vi "Image Processing.vi"(0 "File Path":path=path "C:/General AFM lithography program/Sample.ibw", 1 "Lithography Information":T2(array[cluster])=array7x3944[27608 elements], 2 "Crop?":bool, 3 "Crop Data":T3, 4 "Angle (degrees)":dbl, 5 "error in (no error)":errorcluster, 6 "Size":cluster{"Width":dbl, "Height":dbl}={"Width"=40.0, "Height"=40.0}, 7 "Page":i32=1, 11 "Resolution":i32=1024) -> (14 "Image Out":T4(plugin-control), 15 "Offset":T1={"X Offset (µm)"=-1.2812, "Y Offset (µm)"=5.2969}, 16 "Sample Size":cluster{"Width (µm)":dbl, "Height (µm)":dbl}={"Width (µm)"=40.0, "Height (µm)"=40.0}, 19 "error out":errorcluster)   [LabVIEW 2013]
uses:
  <vilib>/vision/NI_Vision_Development_Module.lvlib
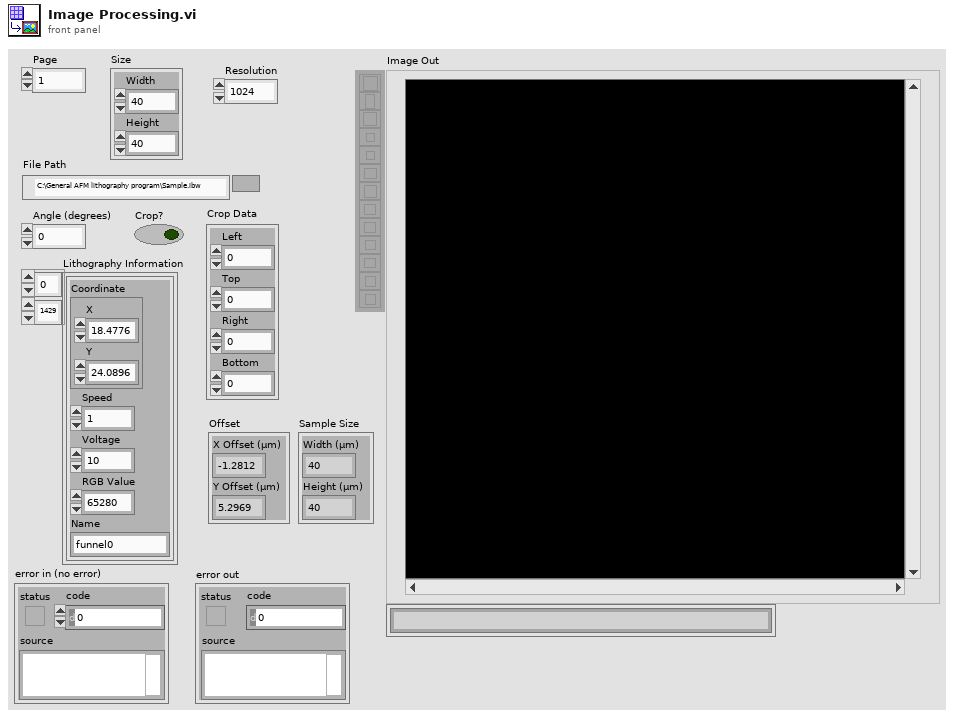
[diagram p1: front panel]
types:
  T1 = cluster{"X Offset (µm)":dbl, "Y Offset (µm)":dbl}
  T2 = cluster{"Coordinate":cluster{"X":dbl, "Y":dbl}, "Speed":dbl, "Voltage":dbl, "RGB Value":i32, "Name":string}[][]
  T3 = cluster{"Left":dbl, "Top":dbl, "Right":dbl, "Bottom":dbl}
  T4 = typedef "IMAQ Image.ctl" = refnum<image>
  T5 = typedef "Image Type" = u32
  T6 = cluster{"Coordinate":cluster{"X":dbl, "Y":dbl}, "Speed":dbl, "Voltage":dbl, "RGB Value":i32, "Name":string}
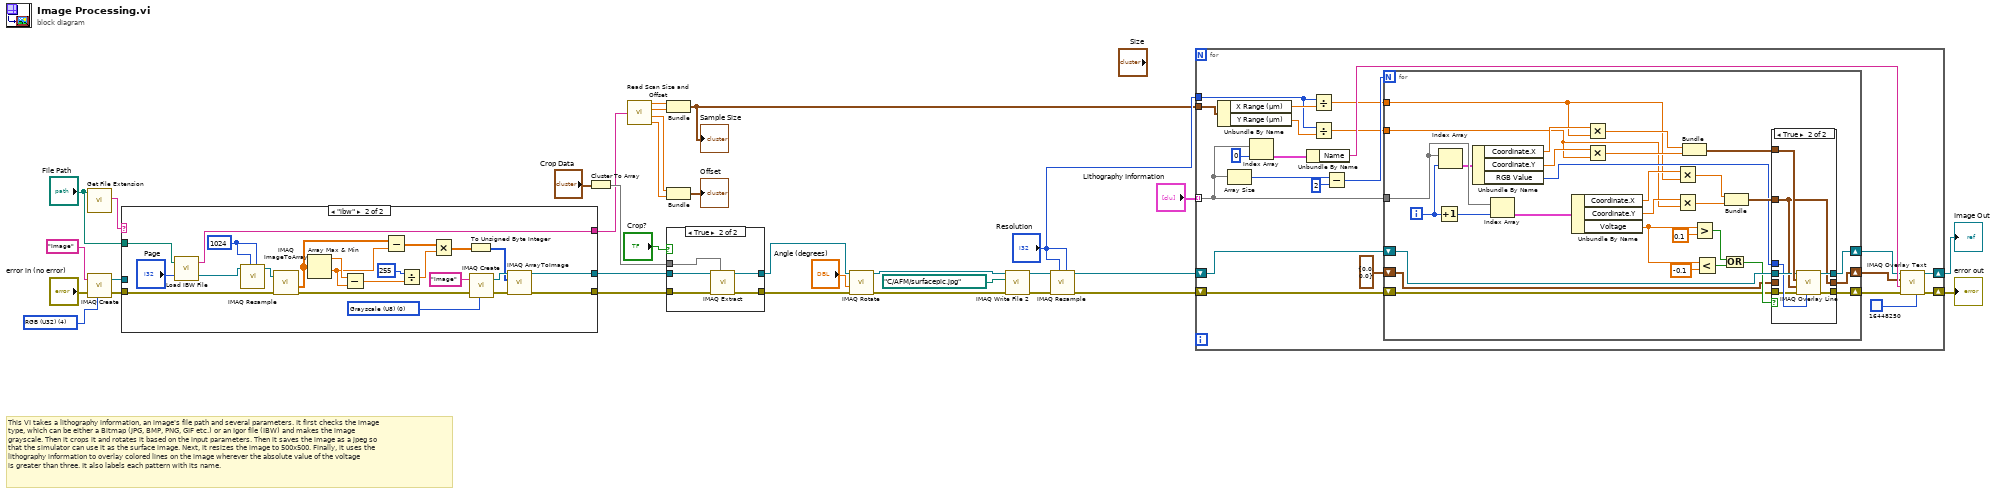
[diagram p0: block diagram]
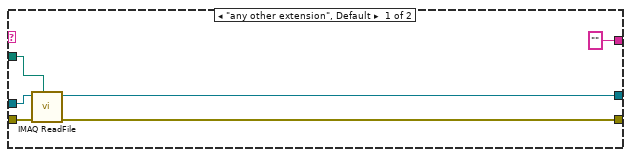
[diagram p2: hidden frame]
diagram:
  w32 = T5 4 items=["Grayscale (U8)", "Grayscale (I16)", "Grayscale (SGL)", "Complex (CSG)", "RGB (U32)", "HSL (U32)", "RGB (U64)", "Grayscale (U16)"] ("Image Type")
  # "This VI takes a lithography information, an image's file path and several parameters. It first checks the image \ntype, which can be either a Bitmap (JPG, BMP, PNG, GIF etc.) or an Igor file (IBW) and makes the image \ngrayscale. Then it crops it and rotates it based on the input parameters. Then it saves the image as a jpeg so \nthat the simulator can use it as the surface image. Next, it resizes the image to 500x500. Finally, it uses the \nlithography information to overlay colored lines on the image wherever the absolute value of the voltage \nis greater than three. It also labels each pattern with its name."
  n1 = call <vilib>:"Get File Extension.vi"("file"="File Path") -> ("lowercase file extension"=w19:string)  [unwired: 7 in, 3 out]
  n2 = call "IMAQ Create"("Image Name"="Image", "Image Type"=w32, "error in (no error)"="error in (no error)") -> ("New Image"=w31:T4, "error out"=w30:errorcluster)  [unwired: 2 in]
  n3 = case shown="\"ibw\"" w19 {
    tunnel: w31 -> [w39 _]
    tunnel: w30 -> [w38 w60]
    tunnel: [w37 w53] -> w29
    tunnel: [w36 w52] -> w28
    tunnel: "File Path" -> [w35 w62]
    tunnel: ["" ("Wave Note") w40] -> w8
    frame "any other extension", Default {
      n4 = call "IMAQ ReadFile"("File Path"=w35, "error in (no error)"=w38, "Image"=w39) -> ("error out"=w36:errorcluster, "Image Out"=w37:T4)  [unwired: 4 in, 3 out]
    }
    frame "ibw" {
      w50 = 1024 ("Y Resolution")
      w57 = T5 0 items=["Grayscale (U8)", "Grayscale (I16)", "Grayscale (SGL)", "Complex (CSG)", "RGB (U32)", "HSL (U32)", "RGB (U64)", "Grayscale (U16)"] ("Image Type")
      n5 = call "Load IBW File.vi"("Page"="Page", "file path (dialog if empty)"=w62) -> ("Image"=w49:T4, "Wave Note"=w40:string)
      n6 = call "IMAQ Resample"("X Resolution"=w50, "Y Resolution"=w50, "Image Src"=w49) -> ("Image Dst Out"=w48:T4)  [unwired: 7 in, 1 out]
      n7 = call "IMAQ ImageToArray"("error in (no error)"=w60, "Image"=w48) -> ("Image Pixels (Float)"=w59:sgl[][], "error out"=w54:errorcluster)  [unwired: 2 in, 3 out]
      n8 = Array Max & Min(array=w59) -> (max value=w47:sgl, min value=w46:sgl)  [unwired: 2 out]
      n9 = Subtract(x=w47, y=w46) -> (x-y=w44:sgl)
      n10 = Subtract(x=w59, y=w46) -> (x-y=w45:sgl[][])
      n11 = Divide(x=255, y=w44) -> (x/y=w42:sgl)
      n12 = Multiply(x=w45, y=w42) -> (x*y=w41:sgl[][])
      n13 = To Unsigned Byte Integer(number=w41) -> (unsigned 8bit integer=w56:u8[][])
      n14 = call "IMAQ Create"("Image Name"="Image", "Image Type"=w57, "error in (no error)"=w54) -> ("New Image"=w58:T4, "error out"=w55:errorcluster)  [unwired: 2 in]
      n15 = call "IMAQ ArrayToImage"("error in (no error)"=w55, "Image Pixels (U8)"=w56, "Image"=w58) -> ("error out"=w52:errorcluster, "Image Out"=w53:T4)  [unwired: 7 in]
    }
  }
  n16 = Cluster To Array(cluster="Crop Data") -> (array=w26:dbl[])
  n17 = call "Read Scan Size and Offset.vi"("Read in the string file"=w8) -> ("X Range (µm)"=w7:dbl, "Y Range (µm)"=w6:dbl, "X Offset (µm)"=w5:dbl, "Y Offset (µm)"=w4:dbl)  [unwired: 4 in]
  n18 = Bundle("X Range (µm)"=w7, "Y Range (µm)"=w6) -> (w1:cluster{"X Range (µm)":dbl, "Y Range (µm)":dbl})  [unwired: 1 in]
  "Sample Size" <- w1
  n19 = Bundle("X Offset (µm)"=w5, "Y Offset (µm)"=w4) -> (→"Offset":T1)  [unwired: 1 in]
  n20 = case shown="True" "Crop?" {
    tunnel: w29 -> [w64 w68]
    tunnel: w28 -> [w63 w67]
    tunnel: w26 -> [_ w69]
    tunnel: [w64 w65] -> w17
    tunnel: [w63 w66] -> w16
    frame False {
    }
    frame True {
      n21 = call "IMAQ Extract"("Optional Rectangle"=w69, "error in (no error)"=w67, "Image Src"=w68) -> ("error out"=w66:errorcluster, "Image Dst Out"=w65:T4)  [unwired: 7 in]
    }
  }
  n22 = call "IMAQ Rotate"("error in (no error)"=w16, "Angle (degrees)"="Angle (degrees)", "Image Src"=w17) -> ("error out"=w13:errorcluster, "Image Dst Out"=w14:T4)  [unwired: 7 in]
  n23 = call-poly "IMAQ Write File 2"("error in (no error)"=w13, "File Path"=path "C:/AFM/surfacepic.jpg", "Image"=w14) -> ("error out"=w11:errorcluster, "Image Out (duplicate)"=w12:T4)  [unwired: 7 in]
  n24 = call "IMAQ Resample"("X Resolution"="Resolution", "Y Resolution"="Resolution", "error in (no error)"=w11, "Image Src"=w12) -> ("error out"=w9:errorcluster, "Image Dst Out"=w10:T4)  [unwired: 6 in]
  n25 = for {
    tunnel: "Lithography Information" -> [w78] mode=indexing
    shift-right: [w80] -> w21
    shift-left: w10 -> [w86]
    shift-right: [w82] -> w24
    shift-left: w9 -> [w88]
    tunnel: "Resolution" -> [w71]
    tunnel: w1 -> [w70]
    n26 = Unbundle By Name(w70) -> ("X Range (µm)"=w73:dbl, "Y Range (µm)"=w72:dbl)
    n27 = Array Size(array=w78) -> (size(s)=w91:i32)
    n28 = Index Array(array=w78, index=0) -> (element=w76:T6)
    n29 = Unbundle By Name(w76) -> ("Name"=w85:string)
    n30 = Divide(x=w71, y=w73) -> (x/y=w75:dbl)
    n31 = Divide(x=w71, y=w72) -> (x/y=w74:dbl)
    n32 = Subtract(x=w91, y=2) -> (x-y=w89:i32)
    n33 = for {
      N: w89 -> [_]
      tunnel: w78 -> [w99]
      shift-right: [w107] -> w81
      shift-left: w86 -> [w116]
      shift-right: [w100] -> w83
      shift-left: w88 -> [w101]
      tunnel: w75 -> [w95]
      shift-right: [w94] -> w79
      shift-left: cluster{dbl, dbl} {0.0, 0.0} -> [w93]
      tunnel: w74 -> [w92]
      i -> [w98]
      n34 = Increment(x=w98) -> (x+1=w117:i32)
      n35 = Index Array(array=w99, index=w98) -> (element=w97:T6)
      n36 = Unbundle By Name(w97) -> ("Coordinate.X"=w121:dbl, "Coordinate.Y"=w120:dbl, "RGB Value"=w108:i32)
      n37 = Index Array(array=w99, index=w117) -> (element=w114:T6)
      n38 = Unbundle By Name(w114) -> ("Coordinate.X"=w112:dbl, "Coordinate.Y"=w113:dbl, "Voltage"=w96:dbl)
      n39 = Multiply(x=w121, y=w95) -> (x*y=w119:dbl)
      n40 = Multiply(x=w120, y=w92) -> (x*y=w118:dbl)
      n41 = Multiply(x=w112, y=w95) -> (x*y=w111:dbl)
      n42 = Multiply(x=w113, y=w92) -> (x*y=w110:dbl)
      n43 = Bundle(w119, w118) -> (w115:cluster{dbl, dbl})  [unwired: 1 in]
      n44 = Greater?(x=w96, y=0.1) -> (0:w104:bool)
      n45 = Less?(x=w96, y=-0.1) -> (x < y?=w103:bool)
      n46 = Or(x=w104, y=w103) -> (x .or. y?=w102:bool)
      n47 = Bundle(w111, w110) -> (w109:cluster{dbl, dbl})  [unwired: 1 in]
      n48 = case shown="True" w102 {
        tunnel: w116 -> [w124 w129]
        tunnel: w115 -> [_ w131]
        tunnel: w109 -> [_ w125]
        tunnel: w108 -> [_ w128]
        tunnel: [w124 w130] -> w107
        tunnel: w101 -> [w123 w127]
        tunnel: [w123 w126] -> w100
        tunnel: [w122 w125] -> w94
        tunnel: w93 -> [w122 _]
        frame False {
        }
        frame True {
          n49 = call "IMAQ Overlay Line"("Color"=w128, "error in (no error)"=w127, "End Point"=w125, "Start Point"=w131, "Image"=w129) -> ("error out"=w126:errorcluster, "Image Out"=w130:T4)  [unwired: 5 in]
        }
      }
    }
    n50 = call "IMAQ Overlay Text"("BG Color (Transparent)"=u32 16448250, "error in (no error)"=w83, "String"=w85, "Origin"=w79, "Image"=w81) -> ("error out"=w82:errorcluster, "Image Out"=w80:T4)  [unwired: 5 in]
  }
  "Image Out" <- w21
  "error out" <- w24
